vi "Size to Connector.vi"(8 "error in (no error)":errorcluster, 11 "Display State In in":T1 caption="State") -> (0 "error out":errorcluster, 3 "Display State In out":T1 caption="State")   [LabVIEW 2020, in "PXISlotGP.xctl"]
uses:
  PXISlotGP.xctl
  State.ctl
  PXISlot XControl/Connector Type.ctl
  AOAIRefs.ctl
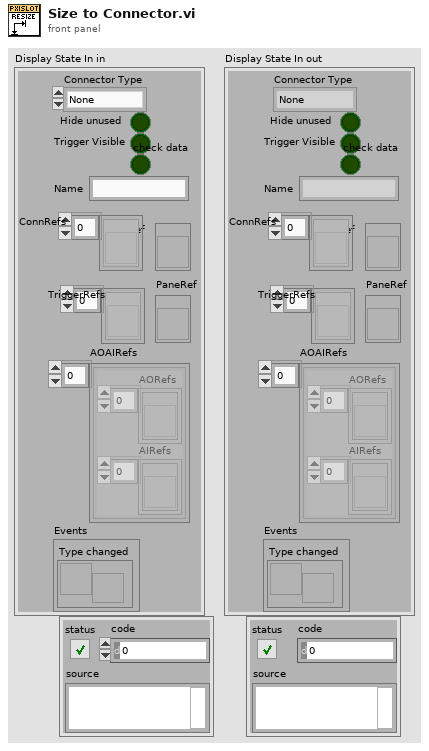
[diagram p1: front panel]
types:
  T1 = typedef "PXISlotGP.xctl/State.ctl" = cluster{"Connector Type":T2, "Hide unused":bool, "Trigger Visible":bool, "TabRef":refnum<vi>, "ConnRefs":refnum<vi>[], "PaneRef":refnum<vi>, "AOAIRefs":T3[], "TriggerRefs":refnum<vi>[], "check data":bool, "Name":string, "Events":cluster{"Type changed":refnum<user-event>}}
  T2 = typedef "Connector Type.ctl" = enum16{"None", "PXI-4461", "BNC-2110", "BNC-2090", "PXIe-4463", "PXIe-4464"}
  T3 = typedef "AOAIRefs.ctl" = cluster{"AORefs":refnum<vi>[], "AIRefs":refnum<vi>[]}
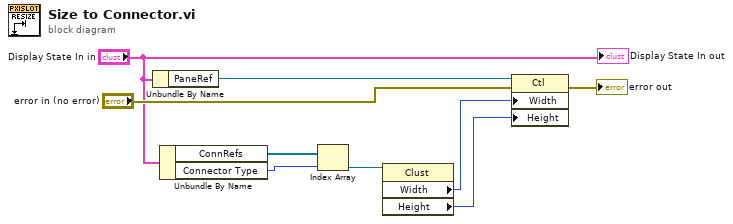
[diagram p0: block diagram]
diagram:
  n1 = Unbundle By Name("Display State In in") -> ("PaneRef"=w3:refnum<vi>)
  n2 = Unbundle By Name("Display State In in") -> ("ConnRefs"=w9:refnum<vi>[], "Connector Type"=w8:T2)
  n3 = Index Array(array=w9, index=w8) -> (element=w7:refnum<vi>)
  n4 = property class="Clust"(reference=w7) -> ("Width"=w2:u32, "Height"=w1:u32)  [unwired: 1 in, 2 out]
  n5 = property class="Ctl"(reference=w3, error in="error in (no error)", "Width"=w2, "Height"=w1) -> (error out=→"error out":errorcluster)  [unwired: 1 out]
  "Display State In out" <- "Display State In in"
